vi "gentec-M-Link.Set Range.vi"(0 "VISA resource In":refnum<visa-resource-name>, 2 "Range":T1 items=["1f", "3f", "10f", "30f", "100f", "300f", "1p", "3p", "10p", "30p", "100p", "300p", "1n", "3n", "10n", "30n", "100n", "300n", "1u", "3u", "10u", "30u", "100u", "300u", "1m", "3m", "10m", "30m", "100m", "300m", "1", "3", "10", "30", "100", "300", "1K", "3K", "10K", "30K", "100K", "300K", "1M", "3M", "10M", "30M", "100M", "300M"], 5 "error in (no error)":errorcluster) -> (11 "Data Read":string, 13 "Read Timeout":bool, 14 "VISA resource Out":refnum<visa-resource-name>, 17 "Success":bool, 19 "error out":errorcluster)   [LabVIEW 2014, in "gentec-M-Link - Driver.lvlib"]
doc: "Data to write: rng<n> where <n> is an integer\n\nSets the instrument range"
uses:
  gentec-M-Link - Driver.lvlib
  Type Defs/gentec-M-Link.Range.ctl
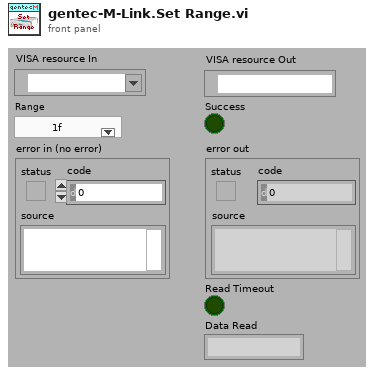
[diagram p1: front panel]
types:
  T1 = typedef "gentec-M-Link - Driver.lvlib/gentec-M-Link.Range.ctl" = u16
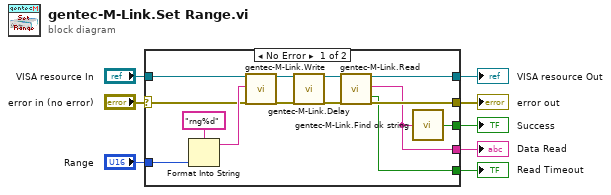
[diagram p0: block diagram]
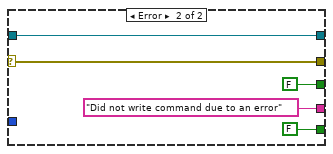
[diagram p2: hidden frame]
diagram:
  n1 = case shown="No Error" "error in (no error)" {
    selector: "error in (no error)" -> [w17 w27]
    tunnel: [w20 w27] -> w7
    tunnel: "VISA resource In" -> [w18 w26]
    tunnel: "Range" -> [w19 _]
    tunnel: [w16 w26] -> w4
    tunnel: [w15 FALSE ("Found")] -> w3
    tunnel: [w13 "Did not write command due to an error" ("Data Read")] -> w2
    tunnel: [w12 FALSE ("Read Timeout")] -> w1
    frame No Error {
      n2 = Format Into String(format string="rng%d", w19) -> (resulting string=w21:string)  [unwired: 2 in, 1 out]
      n3 = call "gentec-M-Link.Write.vi"("VISA resource (In)"=w18, "Data To Write"=w21, "error in (no error)"=w17) -> ("VISA resource (Out)"=w10:refnum<visa-resource-name>, "error out"=w14:errorcluster)  [unwired: 14 in, 1 out]
      n4 = call "gentec-M-Link.Delay.vi"("VISA resource In"=w10, "error in (no error)"=w14) -> ("VISA resource Out"=w9:refnum<visa-resource-name>, "error out"=w11:errorcluster)  [unwired: 16 in]
      n5 = call "gentec-M-Link.Read.vi"("VISA resource (In)"=w9, "error in (no error)"=w11) -> ("VISA resource (Out)"=w16:refnum<visa-resource-name>, "Data Read"=w13:string, "Read Timeout"=w12:bool, "error out"=w20:errorcluster)  [unwired: 13 in, 1 out]
      n6 = call "gentec-M-Link.Find ok string.vi"("string"=w13) -> ("Found"=w15:bool)
    }
    frame Error {
    }
  }
  "error out" <- w7
  "VISA resource Out" <- w4
  "Success" <- w3
  "Data Read" <- w2
  "Read Timeout" <- w1
